vi "Generate STOP command.vi"(8 "Error in":errorcluster) -> (0 "Error out":errorcluster, 3 "Array":u8[](array[numeric]))   [LabVIEW 2020]
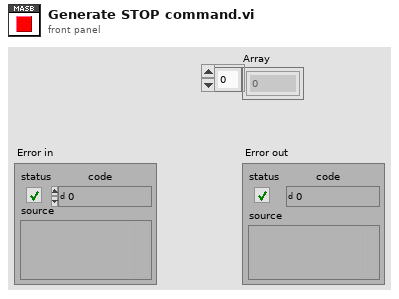
[diagram p1: front panel]
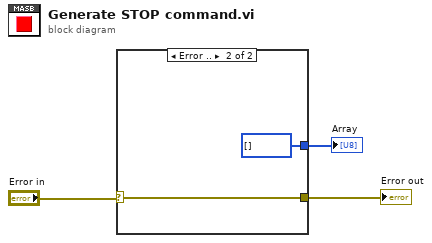
[diagram p0: block diagram]
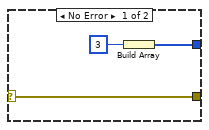
[diagram p2: hidden frame]
diagram:
  n1 = case shown="Error .." "Error in" {
    selector: "Error in" -> [w4 w8]
    tunnel: [w6 u8[] []] -> w3
    tunnel: [w4 w8] -> w1
    frame No Error {
      n2 = Build Array(u8 3) -> (w6:u8[])
    }
    frame Error {
    }
  }
  "Array" <- w3
  "Error out" <- w1
